vi "read CSM log Filter config v1.0.vi"() -> (3 "Rules-v1":T1)   [LabVIEW 2017, in "csm-ini-variable-addon.lvclass"]
uses:
  csm-ini-variable-addon.lvclass
  <userlib>/_NEVSTOP/Communicable State Machine(CSM)/_Support/Typedef/_CSM_GlobalLog Filter Rules - v1.0.ctl
  <userlib>/_NEVSTOP/Communicable State Machine(CSM)/_Support/Typedef/_CSM_GlobalLog_MSG_TYPE.ctl
  <userlib>/_NEVSTOP/Communicable State Machine(CSM)/_Support/Typedef/_CSM_GlobalLog_STATE_TYPE.ctl
  INI-Static-Variable-Support/LabVIEW-Config/LabVIEW-Config.lvclass
  INI-Static-Variable-Support/INI-Static-Variable-Support.lvlib
  <userlib>/_NEVSTOP/Communicable State Machine(CSM)/Communicable State Machine.lvlib
panel:
  out "Key Names":string[](array[string])
  out "error out":errorcluster
  in  "error in (no error)":errorcluster
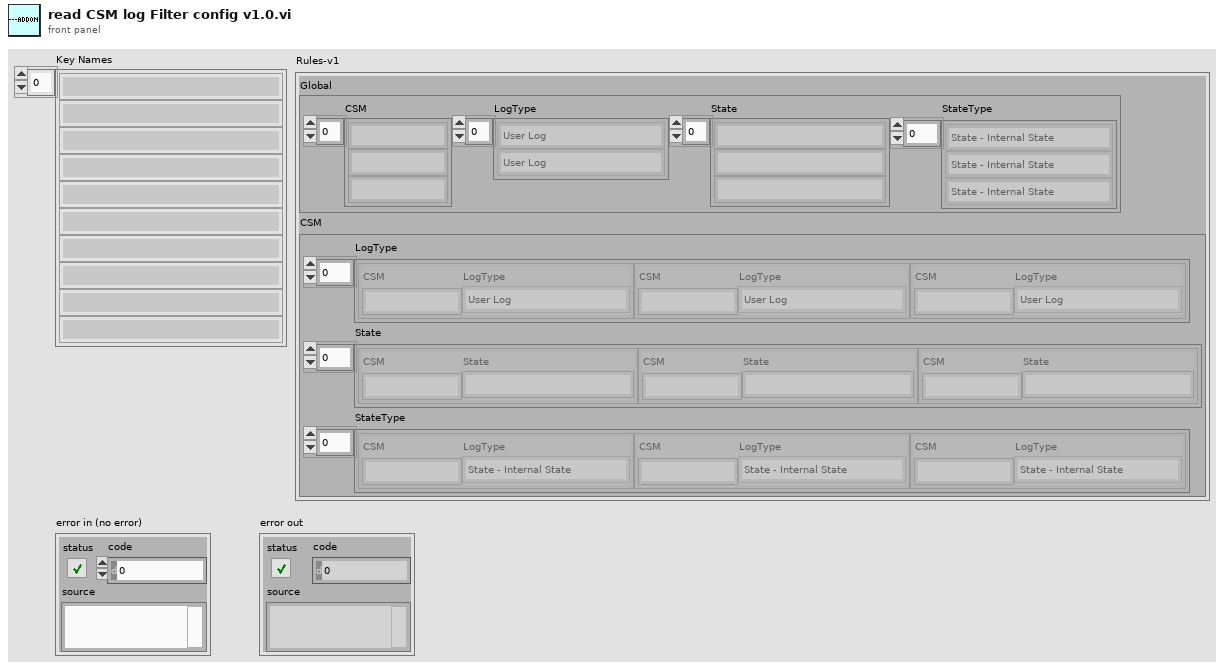
[diagram p1: front panel]
types:
  T1 = typedef "Communicable State Machine.lvlib/_CSM_GlobalLog Filter Rules - v1.0.ctl" = cluster{"Global":cluster{"CSM":string[], "LogType":T2[], "State":string[], "StateType":T3[]}, "CSM":cluster{"LogType":cluster{"CSM":string, "LogType":T2}[], "State":cluster{"CSM":string, "State":string}[], "StateType":cluster{"CSM":string, "LogType":T3}[]}}
  T2 = typedef "Communicable State Machine.lvlib/_CSM_GlobalLog_MSG_TYPE.ctl" = enum16{"User Log", "State Change", "Status", "Interrupt", "Register", "Unregister", "Error Log", "Module Created", "Module Destroyed"}
  T3 = typedef "Communicable State Machine.lvlib/_CSM_GlobalLog_STATE_TYPE.ctl" = enum16{"State - Internal State", "State - External Message", "State - Response", "State - Complete"}
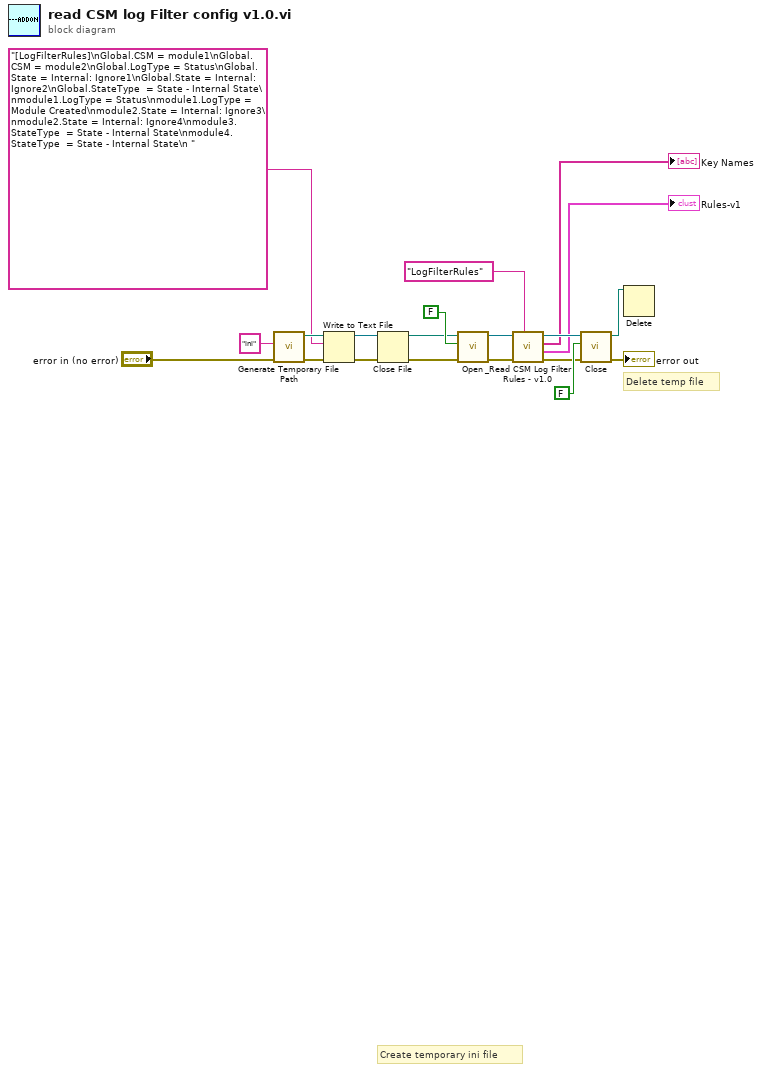
[diagram p0: block diagram]
diagram:
  # "Delete temp file"
  # "Create temporary ini file"
  n1 = call <vilib>:"Generate Temporary File Path.vi"("error in (no error)"="error in (no error)", "Temporary File Extension (tmp)"="ini") -> ("error out"=w17:errorcluster, "Unique Temporary File Path"=w14:path)  [unwired: 8 in]
  n2 = Write to Text File(file (use dialog)=w14, text="[LogFilterRules]\nGlobal.CSM = module1\nGlobal.CSM = module2\nGlobal.LogType = Status\nGlobal.State = Internal: Ignore1\nGlobal.State = Internal: Ignore2\nGlobal.StateType  = State - Internal State\nmodule1.LogType = Status\nmodule1.LogType = Module Created\nmodule2.State = Internal: Ignore3\nmodule2.State = Internal: Ignore4\nmodule3.StateType  = State - Internal State\nmodule4.StateType  = State - Internal State\n ", error in=w17) -> (refnum out=w13:refnum<file>, error out=w15:errorcluster)  [unwired: 1 in, 1 out]
  n3 = Close File(refnum=w13, error in=w15) -> (path=w8:path, error out=w9:errorcluster)
  n4 = call "Open.vi"("error in (no error)"=w9, "Create if not exists? (T)"=FALSE, "Path"=w8) -> ("error out"=w7:errorcluster, "LabVIEW-Config.lvlib:LabVIEW-Config.lvclass"=w5:refnum<class "LabVIEW-Config.lvclass">)  [unwired: 5 in, 2 out]
  n5 = call "_Read CSM Log Filter Rules - v1.0.vi"("Section Name"="LogFilterRules", "error in (no error)"=w7, "LabVIEW-Config.lvlib:LabVIEW-Config.lvclass"=w5) -> ("error out"=w6:errorcluster, "Rules-v1"=→"Rules-v1":T1, "Key Names"=→"Key Names":string[], "Config out"=w4:refnum<class "LabVIEW-Config.lvclass">)  [unwired: 5 in]
  n6 = call "Close.vi"("error in (no error)"=w6, "Write if modified? (T)"=FALSE, "LabVIEW-Config.lvlib:LabVIEW-Config.lvclass"=w4) -> ("error out"=→"error out":errorcluster, "Path"=w11:path)  [unwired: 7 in]
  n7 = Delete(path (use dialog)=w11) -> ()  [unwired: 4 in, 3 out]
